vi "Create Modbus Channels.vi"(8 "error in (no error)":errorcluster, 10 "Array":T3[](array[typedef]), 11 "CD Ref In":T2 format="%.0x") -> (0 "error out":errorcluster, 2 "Channels Refs":T1[](array[typedef]) {"Array of Refs" format="%.0x"})   [LabVIEW 2014, in "Modbus System Explorer.lvlib"]
uses:
  Modbus System Explorer.lvlib
  XML Deserializer/XML VIs/API/Controls/Modbus_Items.ctl
  XML Deserializer/XML VIs/API/Controls/Modbus_Item_Type.ctl
  <vilib>/NI Veristand/Custom Device API/Custom Device Item Ref.ctl
  Shared/Channels Ref.ctl
  <vilib>/NI Veristand/Custom Device API/Custom Device Channel.ctl
  <vilib>/NI Veristand/Custom Device API/Custom Device Channel Type.ctl
  Shared/Modbus GUID Lookup.vi
  <vilib>/NI Veristand/Custom Device API/Custom Device API.lvlib
  Shared/Modbus Shared.lvlib
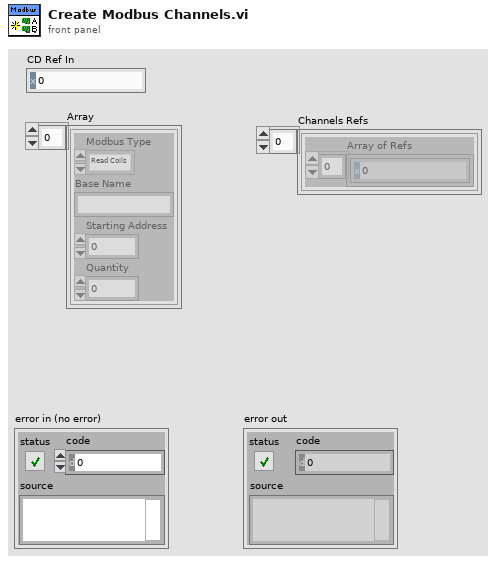
[diagram p1: front panel]
types:
  T1 = typedef "Modbus Shared.lvlib/Channels Ref.ctl" = cluster{"Array of Refs":T2[]}
  T2 = typedef "Custom Device API.lvlib/Custom Device Item Ref.ctl" = u64
  T3 = typedef "Modbus Shared.lvlib/Modbus_Items.ctl" = cluster{"Modbus Type":T4, "Base Name":string, "Starting Address":u16, "Quantity":u16}
  T4 = typedef "Modbus Shared.lvlib/Modbus_Item_Type.ctl" = enum16{"Read Coils", "Read Discrete Inputs", "Read Holding Registers", "Read Input Registers", "Write Multiple Coils", "Write Multiple Holding Registers", "Write Single Coil", "Write Single Holding Register", "Write Multiple Discrete Inputs", "Write Multiple Input Registers"}
  T5 = typedef "Custom Device API.lvlib/Custom Device Channel.ctl" = cluster{"Type":T6, "Units":string, "Default Value":dbl, "Faultable":bool, "Scalable":bool}
  T6 = typedef "Custom Device API.lvlib/Custom Device Channel Type.ctl" = enum16{"Input", "Output"}
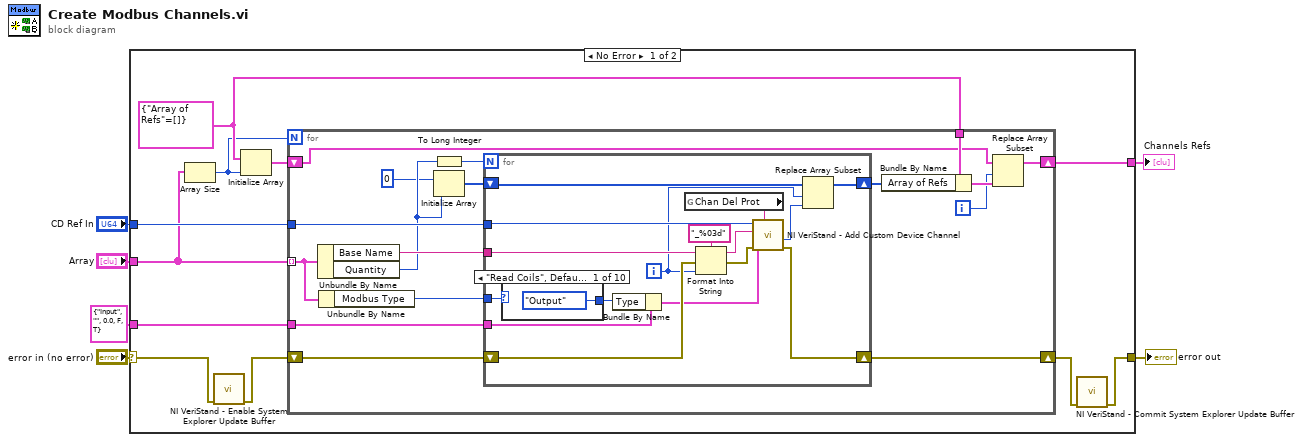
[diagram p0: block diagram]
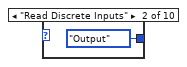
[diagram p2: hidden frame]
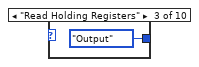
[diagram p3: hidden frame]
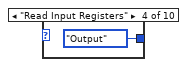
[diagram p4: hidden frame]
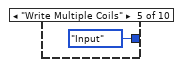
[diagram p5: hidden frame]
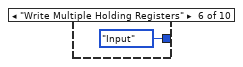
[diagram p6: hidden frame]
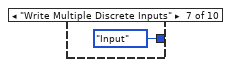
[diagram p7: hidden frame]
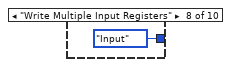
[diagram p8: hidden frame]
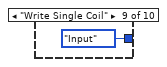
[diagram p9: hidden frame]
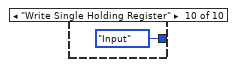
[diagram p10: hidden frame]
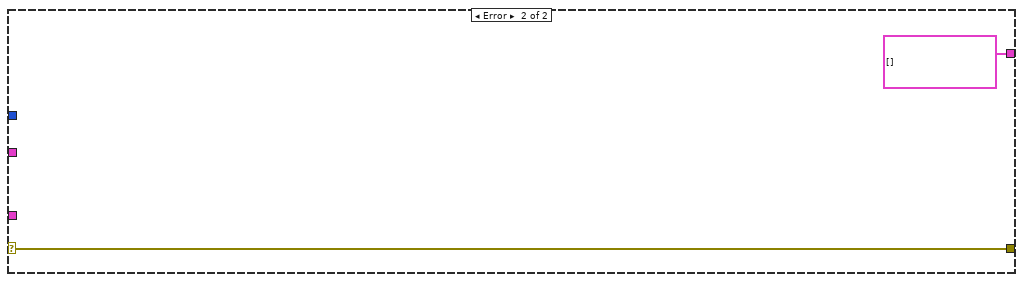
[diagram p11: hidden frame]
diagram:
  n1 = case shown="No Error" "error in (no error)" {
    selector: "error in (no error)" -> [w15 w62]
    tunnel: [w12 w62] -> w5
    tunnel: "CD Ref In" -> [w17 _]
    tunnel: "Array" -> [w11 _]
    tunnel: T5 {"Type"=enum."Input", "Units"="", "Default Value"=0.0, "Faultable"=FALSE, "Scalable"=TRUE} ("Channel") -> [w16 _]
    tunnel: [w8 T1[] []] -> w1
    frame No Error {
      w9 = T1 {"Array of Refs"=[]}
      n2 = Array Size(array=w11) -> (size(s)=w7:i32)
      n3 = call <vilib>:"NI VeriStand - Enable System Explorer Update Buffer.vi"("error in (no error)"=w15) -> ("error out"=w14:errorcluster)  [unwired: 10 in]
      n4 = Initialize Array(w9, w7) -> (w10:T1[])
      n5 = for {
        N: w7 -> [_]
        shift-right: [w31] -> w13
        shift-left: w14 -> [w34]
        tunnel: w11 -> [w29] mode=indexing
        tunnel: w17 -> [w33]
        tunnel: w16 -> [w27]
        shift-right: [w20] -> w8
        shift-left: w10 -> [w21]
        tunnel: w9 -> [w23]
        i -> [w18]
        n6 = Unbundle By Name(w29) -> ("Base Name"=w32:string, "Quantity"=w25:u16)
        n7 = Unbundle By Name(w29) -> ("Modbus Type"=w28:T4)
        n8 = To Long Integer(number=w25) -> (32bit integer=w30:i32)
        n9 = Initialize Array(T2 0 ("Parent Ref out"), w25) -> (w26:T2[])
        n10 = for {
          N: w30 -> [_]
          tunnel: w33 -> [w50]
          tunnel: w32 -> [w47]
          shift-right: [w49] -> w31
          shift-left: w34 -> [w48]
          tunnel: w28 -> [w40]
          tunnel: w27 -> [w42]
          shift-right: [w36] -> w22
          shift-left: w26 -> [w38]
          i -> [w37]
          n11 = case shown="\"Read Coils\", Default" w40 {
            tunnel: [Custom_Device_Channel_Type."Output" ("Type") Custom_Device_Channel_Type."Output" ("Type") Custom_Device_Channel_Type."Output" ("Type") Custom_Device_Channel_Type."Output" ("Type") Custom_Device_Channel_Type."Input" ("Type") Custom_Device_Channel_Type."Input" ("Type") Custom_Device_Channel_Type."Input" ("Type") Custom_Device_Channel_Type."Input" ("Type") Custom_Device_Channel_Type."Input" ("Type") Custom_Device_Channel_Type."Input" ("Type")] -> w39
            frame "Read Coils", Default {
            }
            frame "Read Discrete Inputs" {
            }
            frame "Read Holding Registers" {
            }
            frame "Read Input Registers" {
            }
            frame "Write Multiple Coils" {
            }
            frame "Write Multiple Holding Registers" {
            }
            frame "Write Multiple Discrete Inputs" {
            }
            frame "Write Multiple Input Registers" {
            }
            frame "Write Single Coil" {
            }
            frame "Write Single Holding Register" {
            }
          }
          n12 = Bundle By Name(cluster=w42, "Type"=w39) -> (w41:T5)
          n13 = global read "Modbus GUID Lookup.vi" "Chan Del Prot"() -> (w44:string)
          n14 = Format Into String(format string="_%03d", initial string=w47, error in=w48, w37) -> (resulting string=w43:string, error out=w46:errorcluster)
          n15 = call <vilib>:"NI VeriStand - Add Custom Device Channel.vi"("GUID (Default Channel)"=w44, "error in (no error)"=w46, "Channel"=w41, "Channel Name"=w43, "Parent Ref in"=w50) -> ("error out"=w49:errorcluster, "Channel Ref"=w35:T2)  [unwired: 3 in, 2 out]
          n16 = Replace Array Subset(array=w38, new element=w35, index=w37) -> (w36:T2[])
        }
        n17 = Bundle By Name(cluster=w23, "Array of Refs"=w22) -> (w19:T1)
        n18 = Replace Array Subset(array=w21, new element=w19, index=w18) -> (w20:T1[])
      }
      n19 = call <vilib>:"NI VeriStand - Commit System Explorer Update Buffer.vi"("error in (no error)"=w13) -> ("error out"=w12:errorcluster)  [unwired: 10 in]
    }
    frame Error {
    }
  }
  "error out" <- w5
  "Channels Refs" <- w1
